vi "Get Screen Waveform Data.vi"(8 "error in":errorcluster, 9 "Channel":u8(ring) items=["Channel 1"=1, "Channel 2"=2], 10 "Screen Head":string, 11 "VISA Refnum in":refnum<visa-resource-name>) -> (0 "error out":errorcluster, 2 "Waveform":waveform(dbl), 3 "VISA Refnum out":refnum<visa-resource-name>)   [LabVIEW 2023, in "OWON SDS1022.lvlib"]
uses:
  OWON SDS1022.lvlib
  Horizontal Scale Map.ctl
  Vertical Scale Map.ctl
  Probe Attenuation Map.ctl
  770aa4de-7510-438e-9b4d-035cf8c22fc1.vi
  7861ccd5-a33e-4a01-8da8-89475e14421a.vi
  <vilib>/JDP Science/JSONtext/Find Item.vi
  <vilib>/JDP Science/JSONtext/Next JSON Value.vi
  <vilib>/JDP Science/JSONtext/String Subset.vi
  <vilib>/JDP Science/JSONtext/Parsing/Advance past next JSON Value (inlined COPY).vi
  <vilib>/JDP Science/JSONtext/Parsing/Advance past whitespace.vi
  <vilib>/JDP Science/JSONtext/Parsing/Advance past String.vi
  <vilib>/JDP Science/JSONtext/Parsing/Advance past Number.vi
  <vilib>/JDP Science/JSONtext/Parsing/Advance past Line Ending.vi
  <vilib>/JDP Science/JSONtext/Parsing/Parse Full Path or Item Name.vi
  <vilib>/JDP Science/JSONtext/Parsing/Advance past Array.vi
  <vilib>/JDP Science/JSONtext/Parsing/Advance past Object.vi
  <vilib>/JDP Science/JSONtext/support/Error Cluster From Code.vi
  <vilib>/JDP Science/JSONtext/Offset/Find Item Locations by Path.vi
  <vilib>/JDP Science/JSONtext/JSON text to Variant.vi
  <vilib>/Utility/error.llb/Error Cluster From Error Code.vi
  <vilib>/JDP Science/JSONtext/LVClass Serializer/JSONtext LVClass Serializer.lvclass
  <vilib>/ErrorRing/Error Ring.xnode
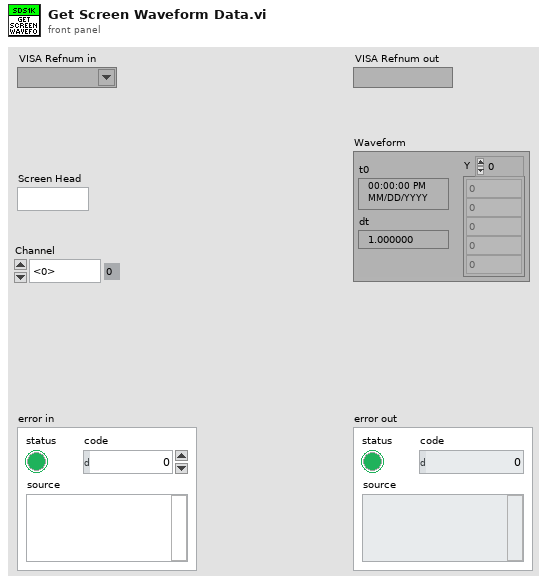
[diagram p1: front panel]
types:
  T1 = typedef "OWON SDS1022.lvlib/Probe Attenuation Map.ctl" = map{string, dbl}
  T2 = typedef "OWON SDS1022.lvlib/Vertical Scale Map.ctl" = map{string, dbl}
  T3 = typedef "OWON SDS1022.lvlib/Horizontal Scale Map.ctl" = map{string, dbl}
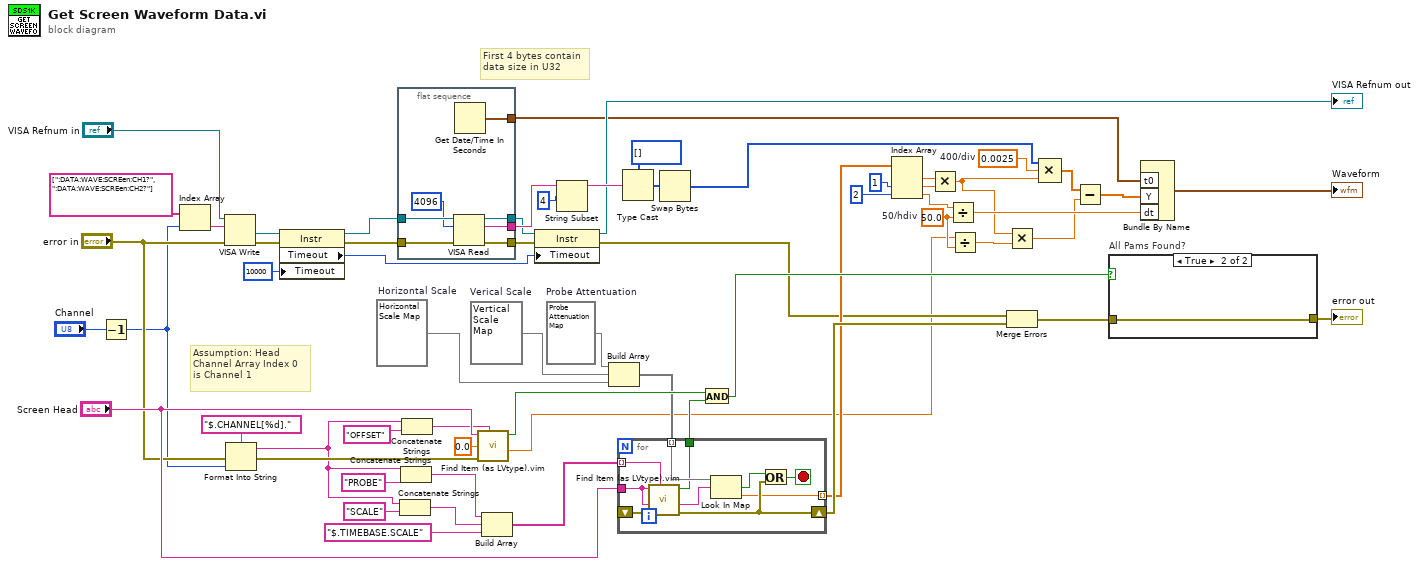
[diagram p0: block diagram]
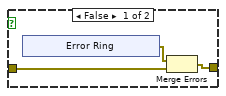
[diagram p2: hidden frame]
diagram:
  w8 = 50.0  # 50/hdiv
  w52 = 0.0025  # 400/div
  w47 = T1 {"0.001X"=0.001, "0.002X"=0.002, "0.005X"=0.005, "0.01X"=0.01, "0.02X"=0.02, "0.05X"=0.05, "0.1X"=0.1, "0.2X"=0.2, "0.5X"=0.5, "1000X"=1000.0, "100X"=100.0, "10X"=10.0, "1X"=1.0, "200X"=200.0, "20X"=20.0, "2X"=2.0, "500X"=500.0, "50X"=50.0, "5X"=5.0}  # Probe Attentuation
  w45 = T2 {"1.00V"=1.0, "10.0V"=10.0, "100mV"=0.1, "10mV"=0.01, "1mv"=0.001, "2.00V"=2.0, "200mV"=0.2, "20mV"=0.02, "2mV"=0.002, "5.00V"=5.0, "500mV"=0.5, "50mV"=0.05, "5mV"=0.005}  # Verical Scale
  w46 = T3 {"1.0ms"=0.001, "1.0s"=1.0, "1.0us"=1e-06, "10.0ns"=1e-08, "1000s"=1000.0, "100ms"=0.1, "100ns"=1e-07, "100s"=100.0, "100us"=0.0001, "10ms"=0.01, "10s"=10.0, "10us"=1e-05, "2.0ms"=0.002, "2.0ns"=2e-09, "2.0s"=2.0, "2.0us"=2e-06, "20.0ns"=2e-08, "200ms"=0.2, "200ns"=2e-07, "200s"=200.0, "200us"=0.0002, "20ms"=0.02, "20s"=20.0, "20us"=2e-05, "5.0ms"=0.005, "5.0ns"=5e-09, "5.0s"=5.0, "5.0us"=5e-06, "50.0ns"=5e-08, "500ms"=0.5, "500ns"=5e-07, "500s"=500.0, "500us"=0.0005, "50ms"=0.05, "50s"=50.0, "50us"=5e-05}  # Horizontal Scale
  # "Assumption: Head\nChannel Array Index 0\nis Channel 1"
  # "First 4 bytes contain\ndata size in U32"
  n1 = Decrement(x="Channel") -> (x-1=w10:u8)
  n2 = Index Array(array=string[] [":DATA:WAVE:SCREen:CH1?", ":DATA:WAVE:SCREen:CH2?"] ("string array"), index=w10) -> (element=w12:string)
  n3 = VISA Write(VISA resource name="VISA Refnum in", write buffer=w12, error in (no error)="error in") -> (VISA resource name out=w25:refnum<visa-resource-name>, error out=w28:errorcluster)  [unwired: 1 out]
  n4 = Format Into String(format string="$.CHANNEL[%d].", error in="error in", w10) -> (resulting string=w41:string, error out=w42:errorcluster)  [unwired: 1 in]
  n5 = property class="Instr"(reference=w25, error in=w28, "Timeout"=u32 10000) -> (reference out=w17:refnum<visa-resource-name>, error out=w16:errorcluster, "Timeout"=w15:u32)
  n6 = flat-sequence {
    tunnel: [w69] -> w22
    tunnel: [w68] -> w18
    tunnel: w17 -> [w67]
    tunnel: w16 -> [w66]
    tunnel: [w65] -> w14
    tunnel: [w64] -> w23
    frame #0 {
      n7 = VISA Read(VISA resource name=w67, byte count=u32 4096, error in (no error)=w66) -> (VISA resource name out=w65:refnum<visa-resource-name>, read buffer=w69:string, error out=w68:errorcluster)  [unwired: 1 out]
      n8 = Get Date/Time In Seconds() -> (seconds since 1Jan1904=w64:timestamp)
    }
  }
  n9 = Concatenate Strings(w41, "SCALE" ("$Path or Item Name")) -> (w34:string)
  n10 = Concatenate Strings(w41, "PROBE" ("$Path or Item Name")) -> (w35:string)
  n11 = Concatenate Strings(w41, "OFFSET" ("$Path or Item Name")) -> (w39:string)
  n12 = call "Find Item (as LVtype).vim"("$Path or Item Name"=w39, "error in (no error)"=w42, "Data Type and Default Value"=0.0, "JSON"="Screen Head") -> ("Data"=w7:dbl, "Found"=w58:bool)  [unwired: 4 in, 2 out]
  n13 = Build Array(w35, w34, "$.TIMEBASE.SCALE" ("$Path or Item Name")) -> (w43:string[])
  n14 = property class="Instr"(reference=w14, error in=w18, "Timeout"=w15) -> (reference out=→"VISA Refnum out":refnum<visa-resource-name>, error out=w50:errorcluster)
  n15 = String Subset(string=w22, offset (0)=4) -> (substring=w29:string)  [unwired: 1 in]
  n16 = Build Array(w47, w45, w46) -> (w48:T3[])
  n17 = for {
    shift-right: [w78] -> w57
    shift-left: _ -> [w79]
    tunnel: w43 -> [w77] mode=indexing
    tunnel: "Screen Head" -> [w76]
    tunnel: w48 -> [w75] mode=indexing
    tunnel: [w71] -> w54 mode=indexing
    tunnel: [w70] -> w59
    stop <- w72 stop-if-true
    n18 = call "Find Item (as LVtype).vim"("$Path or Item Name"=w77, "error in (no error)"=w79, "Data Type and Default Value"=w76, "JSON"=w76) -> ("error out"=w78:errorcluster, "Data"=w74:string, "Found"=w70:bool)  [unwired: 4 in, 1 out]
    n19 = Look In Map(map=w75, key=w74) -> (key not found?=w73:bool, value=w71:dbl)  [unwired: 1 in]
    n20 = Or(x=w73, y=w78) -> (x .or. y?=w72:bool)
  }
  n21 = Type Cast(type=i16[] [], x=w29) -> (*(type *) &x=w20:i16[])
  n22 = Swap Bytes(anything=w20) -> (byte swapped=w61:i16[])
  n23 = And(x=w58, y=w59) -> (x .and. y?=w60:bool)
  n24 = Index Array(array=w54, index #2=1 ("index"), index #3=2 ("index")) -> (element #1=w3:dbl, element #2=w2:dbl, element #3=w1:dbl)  [unwired: 1 in]
  n25 = Multiply(x=w3, y=w2) -> (x*y=w4:dbl)
  n26 = Divide(x=w1, y=w8) -> (x/y=w9:dbl)
  n27 = Divide(x=w7, y=w8) -> (x/y=w6:dbl)
  n28 = Multiply(x=w4, y=w6) -> (x*y=w5:dbl)
  n29 = Merge Errors(w50, w57) -> (w56:errorcluster)
  n30 = Compound Arithmetic op=MULTIPLY(w61, w52, w4) -> (w51:dbl[])
  n31 = Subtract(x=w51, y=w5) -> (x-y=w62:dbl[])
  n32 = case "All Pams Found?" shown="True" w60 {
    tunnel: w56 -> [w81 w88]
    tunnel: [w80 w88] -> w49
    frame False {
      n33 = xnode "Error Ring"() -> ("error out"=w82:errorcluster)
      n34 = Merge Errors(w82, w81) -> (w80:errorcluster)
    }
    frame True {
    }
  }
  "error out" <- w49
  n35 = Bundle By Name("t0"=w23, "Y"=w62, "dt"=w9) -> (→"Waveform":waveform(dbl))  [unwired: 1 in]
